vi "Meas Result Generate TWM InpZ Correction - Generate Files.vi"(8 "error in (no error)":errorcluster, 10 "correction data":T1, 11 "correction file path":path) -> (0 "error out":errorcluster)   [LabVIEW 2020]
doc: "Generate TWM input admittance CSV files from preprocessed measured data."
uses:
  Meas Results TWM Digitizer Correction Data.ctl
  results/Meas Results Correction Structuring Mode.ctl
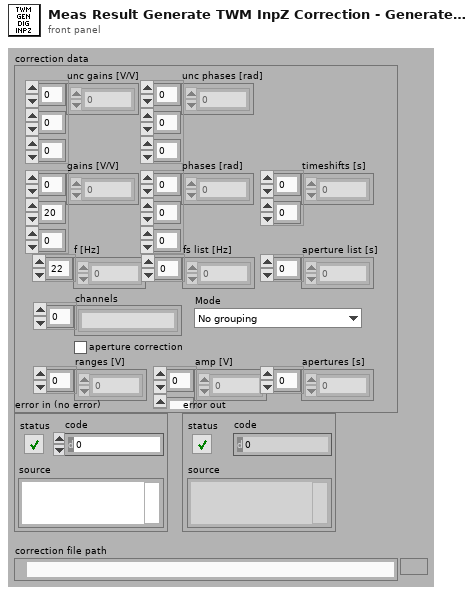
[diagram p1: front panel]
types:
  T1 = typedef "Meas Results TWM Digitizer Correction Data.ctl" = cluster{"gains [V/V]":dbl[][][], "phases [rad]":dbl[][][], "timeshifts [s]":dbl[][], "f [Hz]":dbl[], "fs list [Hz]":dbl[], "aperture list [s]":dbl[], "channels":string[], "Mode":T2, "aperture correction":bool, "ranges [V]":dbl[], "amp [V]":dbl[][], "apertures [s]":dbl[], "unc gains [V/V]":dbl[][][], "unc phases [rad]":dbl[][][]}
  T2 = typedef "Meas Results Correction Structuring Mode.ctl" = enum16{"No grouping", "Group by apertures (3458A)", "Group by fs (generic digitizer)"}
  T3 = enum16{"open", "replace", "create", "open or create", "replace or create", "replace or create with confirmation"}
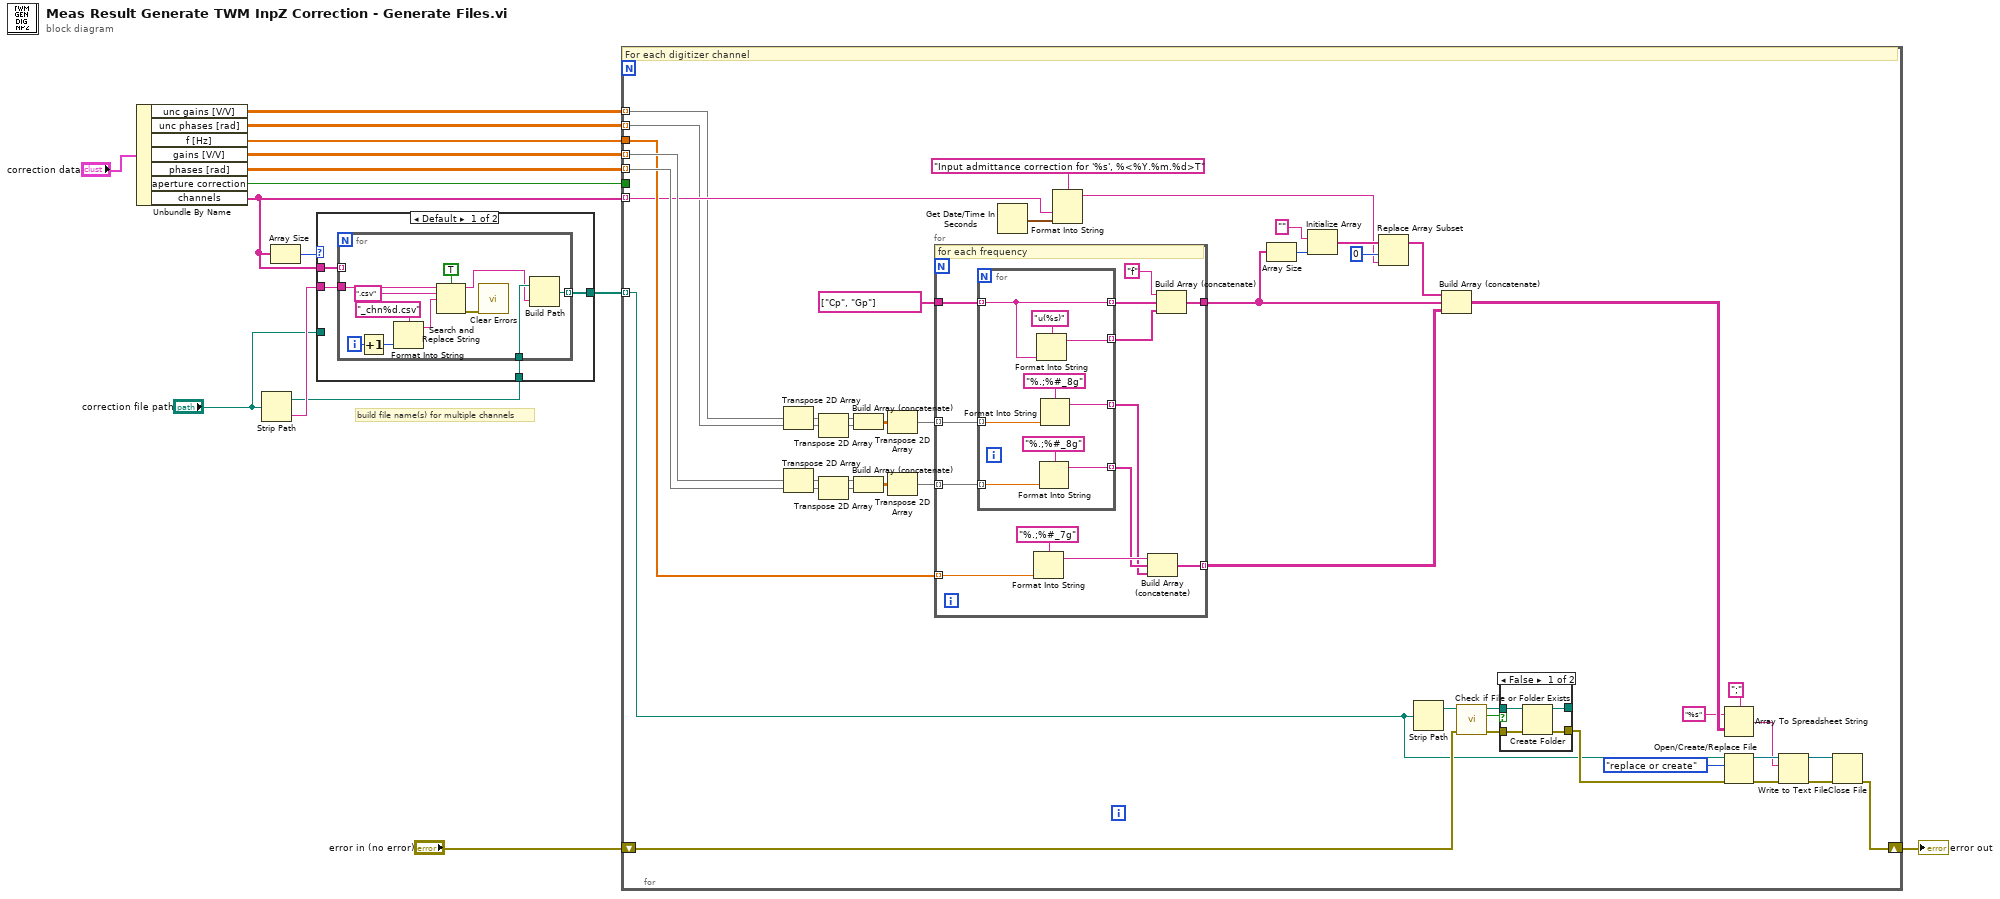
[diagram p0: block diagram]
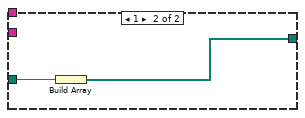
[diagram p2: hidden frame]
diagram:
  # "build file name(s) for multiple channels"
  n1 = Unbundle By Name("correction data") -> ("unc gains [V/V]"=w2:dbl[][][], "unc phases [rad]"=w1:dbl[][][], "f [Hz]"=w12:dbl[], "gains [V/V]"=w11:dbl[][][], "phases [rad]"=w10:dbl[][][], "aperture correction"=w14:bool, "channels"=w7:string[])
  n2 = Strip Path(path="correction file path") -> (stripped path=w5:path, name=w6:string)
  n3 = Array Size(array=w7) -> (size(s)=w8:i32)
  n4 = case shown="Default" w8 {
    tunnel: w7 -> [w19 _]
    tunnel: w6 -> [w18 _]
    tunnel: [w16 w32] -> w3
    tunnel: w5 -> [w17 _]
    tunnel: "correction file path" -> [_ w31]
    frame Default {
      n5 = for {
        tunnel: w19 -> [_] mode=indexing
        tunnel: w18 -> [w30]
        tunnel: w17 -> [w22]
        tunnel: [w20] -> w16 mode=indexing
        i -> [w27]
        n6 = Increment(x=w27) -> (x+1=w26:i32)
        n7 = Format Into String(format string="_chn%d.csv", w26) -> (resulting string=w24:string)  [unwired: 2 in, 1 out]
        n8 = Search and Replace String(case sensitive?=TRUE ("ignore case? (F)"), input string=w30, search string=".csv", replace string=w24) -> (result string=w21:string, error out=w23:errorcluster)  [unwired: 4 in, 2 out]
        n9 = call <vilib>:"Clear Errors.vi"("error in (no error)"=w23) -> ()  [unwired: 5 in, 2 out]
        n10 = Build Path(base path=w22, name or relative path=w21) -> (appended path=w20:path)
      }
    }
    frame 1 {
      n11 = Build Array(w31) -> (w32:path[])
    }
  }
  n12 = for {
    tunnel: w7 -> [w43] mode=indexing
    tunnel: w14 -> [_]
    shift-right: [w44] -> w13
    shift-left: "error in (no error)" -> [w51]
    tunnel: w10 -> [w47] mode=indexing
    tunnel: w12 -> [w46]
    tunnel: w11 -> [w48] mode=indexing
    tunnel: w3 -> [w42] mode=indexing
    tunnel: w2 -> [w34] mode=indexing
    tunnel: w1 -> [w33] mode=indexing
    # "For each digitizer channel"
    n13 = Transpose 2D Array(2D array=w34) -> (transposed array=w37:dbl[][])
    n14 = Transpose 2D Array(2D array=w48) -> (transposed array=w41:dbl[][])
    n15 = Transpose 2D Array(2D array=w33) -> (transposed array=w38:dbl[][])
    n16 = Transpose 2D Array(2D array=w47) -> (transposed array=w40:dbl[][])
    n17 = Build Array (concatenate)(w37, w38) -> (w36:dbl[][])
    n18 = Build Array (concatenate)(w41, w40) -> (w45:dbl[][])
    n19 = Transpose 2D Array(2D array=w36) -> (transposed array=w35:dbl[][])
    n20 = Transpose 2D Array(2D array=w45) -> (transposed array=w39:dbl[][])
    n21 = for {
      tunnel: w46 -> [w91] mode=indexing
      tunnel: w39 -> [w93] mode=indexing
      tunnel: w35 -> [w90] mode=indexing
      tunnel: [w86] -> w66 mode=indexing
      tunnel: string[] ["Cp", "Gp"] ("header") -> [w85]
      tunnel: [w81] -> w67
      # "for each frequency"
      n22 = for {
        tunnel: w93 -> [w101] mode=indexing
        tunnel: w90 -> [w99] mode=indexing
        tunnel: [w98] -> w87 mode=indexing
        tunnel: [w97] -> w88 mode=indexing
        tunnel: w85 -> [w95] mode=indexing
        tunnel: [w95] -> w83 mode=indexing
        tunnel: [w94] -> w82 mode=indexing
        n23 = Format Into String(format string="u(%s)", w95) -> (resulting string=w94:string)  [unwired: 2 in, 1 out]
        n24 = Format Into String(format string="%.;%#_8g", w101) -> (resulting string=w97:string)  [unwired: 2 in, 1 out]
        n25 = Format Into String(format string="%.;%#_8g", w99) -> (resulting string=w98:string)  [unwired: 2 in, 1 out]
      }
      n26 = Format Into String(format string="%.;%#_7g", w91) -> (resulting string=w89:string)  [unwired: 2 in, 1 out]
      n27 = Build Array (concatenate)(w89, w88, w87) -> (w86:string[])
      n28 = Build Array (concatenate)("f", w83, w82) -> (w81:string[])
    }
    n29 = Get Date/Time In Seconds() -> (seconds since 1Jan1904=w74:timestamp)
    n30 = Format Into String(format string="Input admittance correction for '%s', %<%Y.%m.%d>T", w43, w74) -> (resulting string=w50:string)  [unwired: 2 in, 1 out]
    n31 = Array Size(array=w67) -> (size(s)=w72:i32)
    n32 = Initialize Array("", w72) -> (w70:string[])
    n33 = Replace Array Subset(array=w70, new element=w50, index=0) -> (w68:string[])
    n34 = Strip Path(path=w42) -> (stripped path=w62:path)  [unwired: 1 out]
    n35 = Build Array (concatenate)(w68, w67, w66) -> (w60:string[][])
    n36 = call <vilib>:"Check if File or Folder Exists.vi"("error in (no error)"=w51, "path"=w62) -> ("error out"=w63:errorcluster, "file or folder exists?"=w65:bool, "dup path"=w64:path)  [unwired: 7 in]
    n37 = case shown="False" w65 {
      tunnel: w64 -> [w78 w79]
      tunnel: [w77 w79] -> _
      tunnel: w63 -> [w76 w80]
      tunnel: [w75 w80] -> w57
      frame False {
        n38 = Create Folder(path (use dialog)=w78, error in=w76) -> (created path=w77:path, error out=w75:errorcluster)  [unwired: 1 in, 1 out]
      }
      frame True {
      }
    }
    n39 = Array To Spreadsheet String(delimiter (Tab)=";", array=w60, 3:"%s" ("format string")) -> (spreadsheet string=w54:string)
    n40 = Open/Create/Replace File(file path (use dialog)=w42, error in=w57, operation (0:open)=T3."replace or create") -> (refnum out=w55:refnum<file>, error out=w56:errorcluster)  [unwired: 3 in, 1 out]
    n41 = Write to Text File(file (use dialog)=w55, text=w54, error in=w56) -> (refnum out=w52:refnum<file>, error out=w53:errorcluster)  [unwired: 1 in, 1 out]
    n42 = Close File(refnum=w52, error in=w53) -> (error out=w44:errorcluster)  [unwired: 1 out]
  }
  "error out" <- w13
